vi "Init.vi"(10 "jettl":refnum<class "jettl.lvclass">) -> (3 "Last Ack Created Msg Strategy out":refnum<class "Last Ack Created Msg Strategy.lvclass">)   [LabVIEW 2021, in "jettl.lvlib" / "Last Ack Created Msg Strategy.lvlib" / "Last Ack Created Msg Strategy.lvclass"]
uses:
  Last Ack Created Msg Strategy.lvclass
  jettl/jettl.lvclass
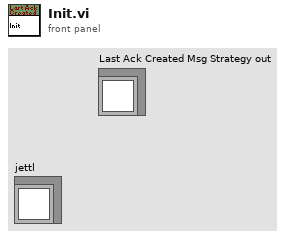
[diagram p1: front panel]
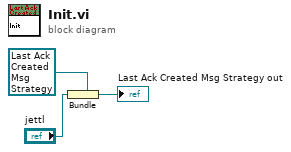
[diagram p0: block diagram]
diagram:
  n1 = Bundle "Bundle"(cluster=refnum<class "Last Ack Created Msg Strategy.lvclass"> refnum ("Last Ack Msg in"), "jettl") -> (→"Last Ack Created Msg Strategy out":refnum<class "Last Ack Created Msg Strategy.lvclass">)
